vi "Get Counts from Datatype.vi"(8 "error in (no error)":errorcluster, 11 "Type":variant) -> (0 "error out":errorcluster, 3 "Terminal Counts":T1)   [LabVIEW 2026, in "VILab.lvlib"]
uses:
  VILab.lvlib
  CTLs/Terminal Counts.ctl
  <vilib>/Utility/Data Type/NI_Data Type.lvlib
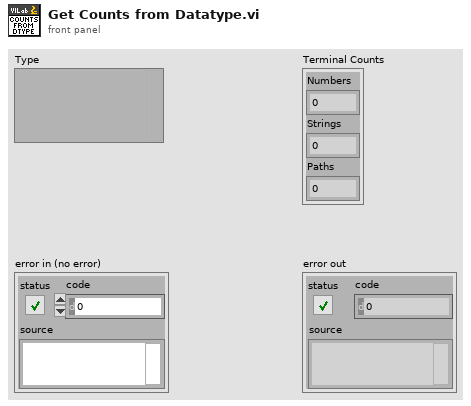
[diagram p1: front panel]
types:
  T1 = typedef "VILab.lvlib/Terminal Counts.ctl" = cluster{"Numbers":u32, "Strings":u32, "Paths":u32}
  T2 = typedef "NI_Data Type.lvlib/Data Type.ctl" = enum8{"Invalid Type", "Void", "I8", "I16", "I32", "I64", "U8", "U16", "U32", "U64", "Single Float", "Double Float", "Extended Float", "Single Complex", "Double Complex", "Extended Complex", "Enum U8", "Enum U16", "Enum U32", "Enum U64", "Single Float With Unit", "Double Float With Unit", "Extended Float With Unit", "Single Complex with Unit", "Double Complex with Unit", "Extended Complex with Unit", "Boolean", "String", "Path", "Picture", "Tag", "Array", "Cluster", "Variant", "LV Variant", "Waveform", "Timestamp", "Digital Waveform", "Digital Data", "ExpressData", "Refnum", "External Data", "VI", "Poly VI", "LabVIEW Class Instance", "Fixed Point", "Set Collection", "Map Collection"}
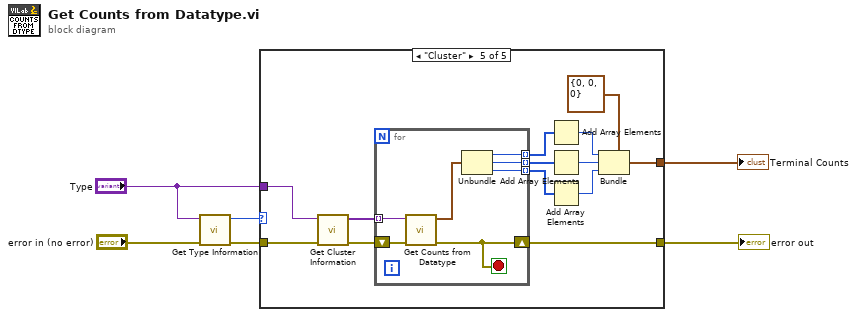
[diagram p0: block diagram]
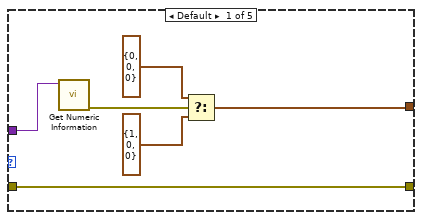
[diagram p2: hidden frame]
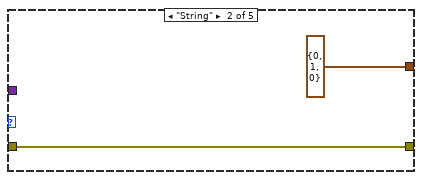
[diagram p3: hidden frame]
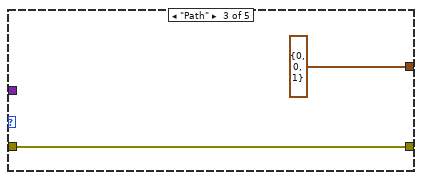
[diagram p4: hidden frame]
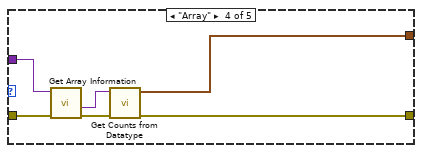
[diagram p5: hidden frame]
diagram:
  n1 = call <vilib>:"Get Type Information.vi"("error in (no error)"="error in (no error)", "variant"="Type") -> ("error out"=w2:errorcluster, "type"=w6:T2)  [unwired: 5 in, 3 out]
  n2 = case shown="\"Cluster\"" w6 {
    tunnel: "Type" -> [w12 _ _ w22 w35]
    tunnel: [w10 T1 {"Numbers"=0, "Strings"=1, "Paths"=0} ("Terminal Counts") T1 {"Numbers"=0, "Strings"=0, "Paths"=1} ("Terminal Counts") w20 w26] -> w3
    tunnel: w2 -> [w7 w13 w15 w19 w25]
    tunnel: [w7 w13 w15 w17 w24] -> w1
    frame Default {
      n3 = call <vilib>:"Get Numeric Information.vi"("variant"=w12) -> ("error out"=w11:errorcluster)  [unwired: 7 in, 3 out]
      n4 = Select(t=T1 {"Numbers"=0, "Strings"=0, "Paths"=0} ("Terminal Counts"), s=w11, f=T1 {"Numbers"=1, "Strings"=0, "Paths"=0} ("Terminal Counts")) -> (s? t:f=w10:T1)
    }
    frame "String" {
    }
    frame "Path" {
    }
    frame "Array" {
      n5 = call <vilib>:"Get Array Information.vi"("error in (no error)"=w19, "variant"=w22) -> ("error out"=w18:errorcluster, "array element data type"=w21:variant)  [unwired: 6 in, 2 out]
      n6 = call "Get Counts from Datatype.vi"("error in (no error)"=w18, "Type"=w21) -> ("error out"=w17:errorcluster, "Terminal Counts"=w20:T1)  [unwired: 8 in]
    }
    frame "Cluster" {
      n7 = call <vilib>:"Get Cluster Information.vi"("error in (no error)"=w25, "variant"=w35) -> ("error out"=w33:errorcluster, "cluster elements"=w34:variant[])  [unwired: 8 in]
      n8 = for {
        tunnel: w34 -> [w42] mode=indexing
        shift-right: [w40] -> w24
        shift-left: w33 -> [w41]
        tunnel: [w39] -> w32 mode=indexing
        tunnel: [w38] -> w31 mode=indexing
        tunnel: [w37] -> w30 mode=indexing
        stop <- w40 stop-if-true
        n9 = call "Get Counts from Datatype.vi"("error in (no error)"=w41, "Type"=w42) -> ("error out"=w40:errorcluster, "Terminal Counts"=w36:T1)  [unwired: 8 in]
        n10 = Unbundle(w36) -> ("Numbers"=w39:u32, "Strings"=w38:u32, "Paths"=w37:u32)
      }
      n11 = Add Array Elements(numeric array=w32) -> (sum=w29:u32)
      n12 = Add Array Elements(numeric array=w31) -> (sum=w28:u32)
      n13 = Add Array Elements(numeric array=w30) -> (sum=w27:u32)
      n14 = Bundle(cluster=T1 {"Numbers"=0, "Strings"=0, "Paths"=0} ("Terminal Counts"), "Numbers"=w29, "Strings"=w28, "Paths"=w27) -> (w26:T1)
    }
  }
  "error out" <- w1
  "Terminal Counts" <- w3
